vi "Refnum Names.vi"() -> ()   [LabVIEW 2014]
panel:
  out "Tote too far Right (Inside)":string="Tote too far Right (Inside)"
  out "Tote too far Right (Outside)":string="Tote too far Right (Outside)"
  out "Tote too far Left (Inside)":string="Tote too far Left (Inside)"
  out "Tote too far Left (Outside)":string="Tote too far Left (Outside)"
  out "Lift - Position 3 (AUTO)":string="Lift - Position 3 (AUTO)"
  out "Left Arm Twister":string="Left Arm Twister"
  out "IO Board 2":string="IO Board 2"
  out "IO Board 1":string="IO Board 1"
  out "Tote in Position/Ready to Lift":string="Tote in Position or Ready to Lift"
  out "Lift - Position 5":string="Lift - Position 5"
  out "Lift - Position 4":string="Lift - Position 4"
  out "Lift - Position 3":string="Lift - Position 3"
  out "Lift - Position 2":string="Lift - Position 2"
  out "Swerve Sensors":string="Swerve Sensors"
  out "Grabber Solenoid":string="Grabber Solenoid"
  out "Scissors":string="Scissors"
  out "Arms":string="Arms"
  out "Can Solenoid":string="Can Solenoid"
  out "Left Back Swivel Position Encoder":string="Left Back Swivel Position Encoder "
  out "Right Back Swivel Position Encoder":string="Right Back Swivel Position Encoder"
  out "Left Front Swivel Position Encoder":string="Left Front Swivel Position Encoder"
  out "Right Front Swivel Position Encoder":string="Right Front Swivel Position Encoder"
  out "Gyro":string="Gyro"
  out "Lift Encoder":string="Lift Encoder"
  out "Lift - Position 1":string="Lift - Position 1"
  out "Drive Encoder":string="Drive Encoder"
  out "Lift Motor":string="Lift Motor"
  out "Right Arm Twister":string="Right Arm Twister"
  out "Joystick":string="Joystick"
  out "Test Gamepad":string="Test Gamepad"
  out "Left Rear Rotator":string="Left Rear Rotator"
  out "Left Rear Wheel":string="Left Rear Wheel"
  out "Left Front Rotator":string="Left Front Rotator"
  out "Left Front Wheel":string="Left Front Wheel"
  out "Right Rear Rotator":string="Right Rear Rotator"
  out "Right Rear Wheel":string="Right Rear Wheel"
  out "Right Front Rotator":string="Right Front Rotator"
  out "Right Front Wheel":string="Right Front Wheel"
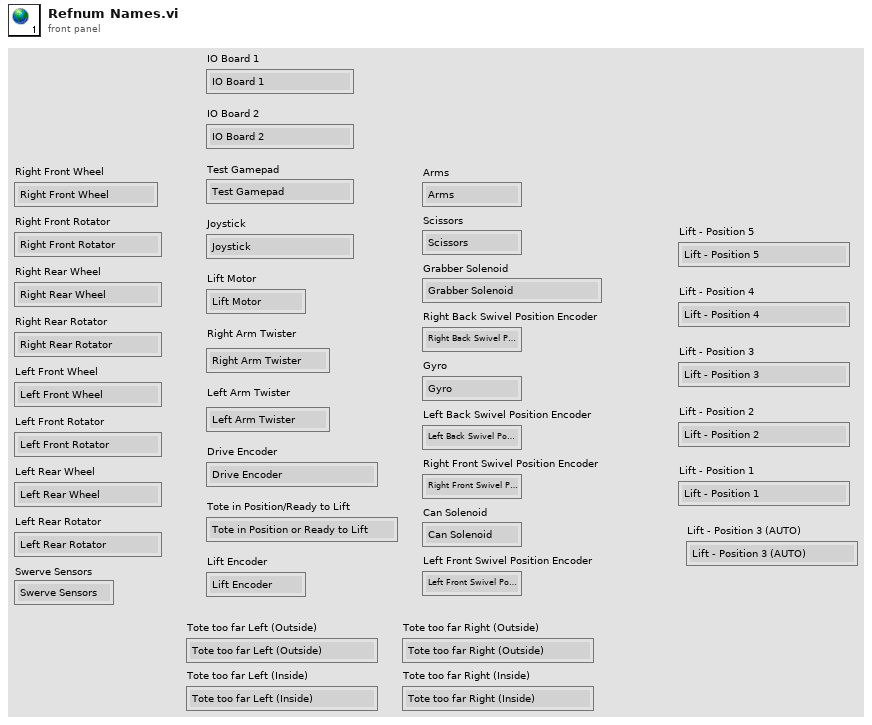
[diagram p1: front panel]
diagram:
